vi "GetType.vi"(8 "error in (no error)":errorcluster, 11 "Stop Pattern Msg":refnum<class "Stop Pattern Msg.lvclass">) -> (0 "error out":errorcluster, 2 "Data Sample":variant, 3 "Stop Pattern Msg":refnum<class "Stop Pattern Msg.lvclass">)   [LabVIEW 2015, in "CS++PPG.lvlib" / "Stop Pattern Msg.lvclass"]
uses:
  Stop Pattern Msg.lvclass
  Stop Pattern Msg.lvclass/Stop Pattern Msg.ctl
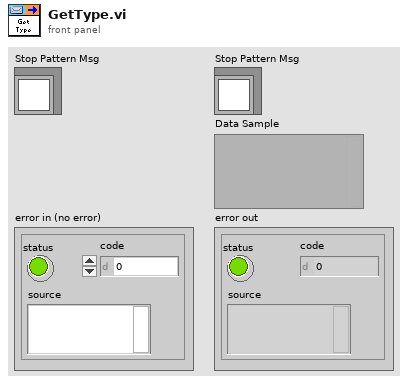
[diagram p1: front panel]
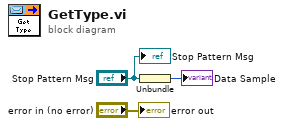
[diagram p0: block diagram]
diagram:
  n1 = Unbundle("Stop Pattern Msg") -> (→"Data Sample":i32)
  "error out" <- "error in (no error)"
  "Stop Pattern Msg" <- "Stop Pattern Msg"
